vi "Write Kernel Size.vi"(8 "error in (no error)":errorcluster, 10 "Kernel Size":enum16{"3x3", "5x5", "3x5", "5x3"}(ring), 11 "Std. Deviation in":refnum<class "Std. Deviation.lvclass">) -> (0 "error out":errorcluster, 3 "Std. Deviation out":refnum<class "Std. Deviation.lvclass">)   [LabVIEW 2015, in "Std. Deviation.lvclass"]
uses:
  Std. Deviation.lvclass
  Std. Deviation.lvclass/Std. Deviation.ctl
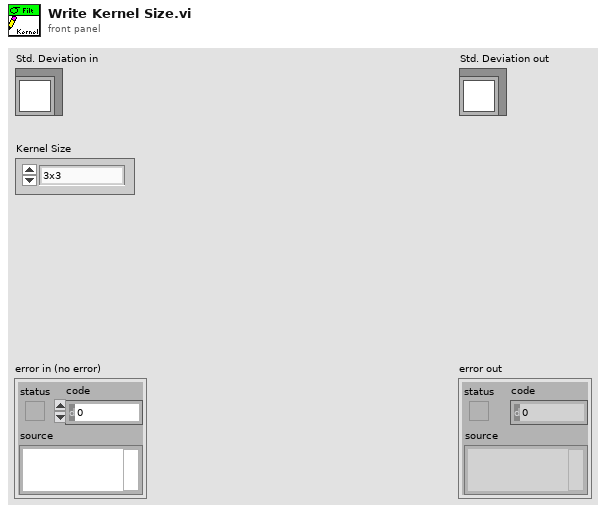
[diagram p1: front panel]
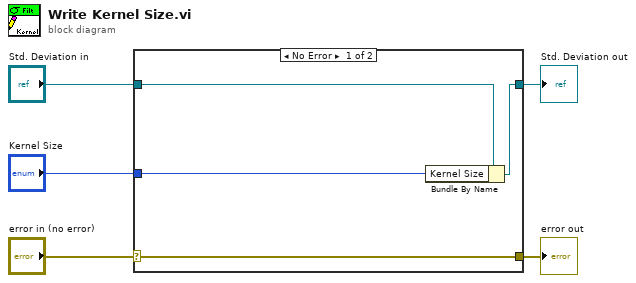
[diagram p0: block diagram]
diagram:
  n1 = case shown="No Error" "error in (no error)" {
    selector: "error in (no error)" -> [w9 w10]
    tunnel: [w9 w10] -> w4
    tunnel: [w7 w11] -> w2
    tunnel: "Std. Deviation in" -> [w8 w11]
    tunnel: "Kernel Size" -> [w6 _]
    frame No Error {
      n2 = Bundle By Name(cluster=w8, "Kernel Size"=w6) -> (w7:refnum<class "Std. Deviation.lvclass">)
    }
    frame Error {
    }
  }
  "error out" <- w4
  "Std. Deviation out" <- w2
